vi "MultiSend.vi"() -> ()   [LabVIEW 2019]
uses:
  ByteGSAPIBase/ByteGSAPIBase.lvclass
  TypeDef/ChannelInfo.ctl
  ByteGSAPIBase/LimsTestStep/acquisitions.ctl
  ByteGSAPIBase/UpdateChannelsList/fields.ctl
  <vilib>/Bytelabs/ByteSimpleQ/ByteSimpleQ/ByteSimpleQ.lvlib
panel:
  in  "Start/Stop":bool
  out "Running":bool
  out "error out":errorcluster
  in  "error in (no error)":errorcluster
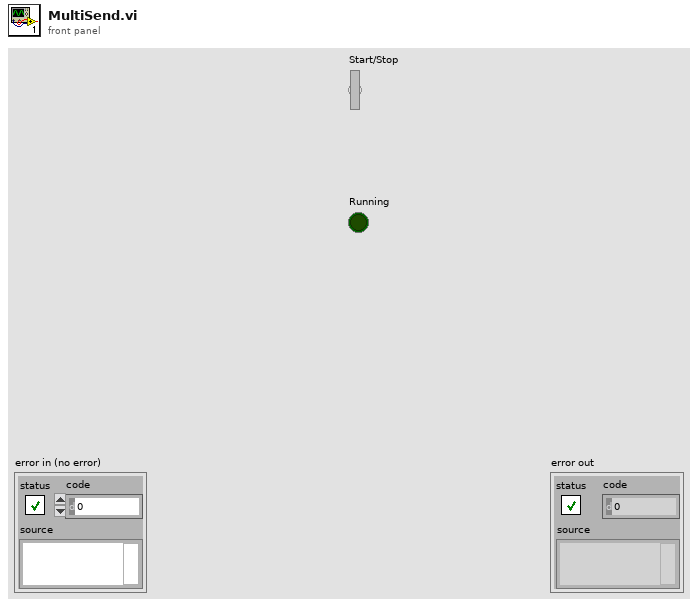
[diagram p1: front panel]
types:
  T1 = typedef "ByteGSWebAPI.lvlib/ByteGSAPIBase.lvclass/acquisitions.ctl" = cluster{"tags":cluster{"step_id":i32, "test_slug":string, "asset_slug":string}, "acquisitions":cluster{"timestamp":string, "fields":cluster{"name":string, "value":dbl}[]}[]}
  T2 = typedef "ChannelInfo.ctl" = cluster{"Tag":string, "HW Resource":string, "Raw":dbl}
  T3 = cluster{"ByteGSAPIBase in":refnum<class "ByteGSAPIBase.lvclass">, "fields":string[][], "Acquisitions":T1, "Info":T2[]}
  T4 = cluster{"ByteGSAPIBase in":refnum<class "ByteGSAPIBase.lvclass">, "queue out":refnum<queue>, "Slug":string, "fields":string[][]}
  T5 = typedef "ByteGSWebAPI.lvlib/ByteGSAPIBase.lvclass/fields.ctl" = cluster{"asset_slug":string, "fields":string[]}
  T6 = cluster{"ByteGSAPIBase out":refnum<class "ByteGSAPIBase.lvclass">, "fields":string[], "Slug":string}
  T7 = cluster{"timestamp":string, "fields":cluster{"name":string, "value":dbl}[]}
  T8 = cluster{"timestamp":string, "fields":cluster{"name":string, "value":dbl}[]}[]
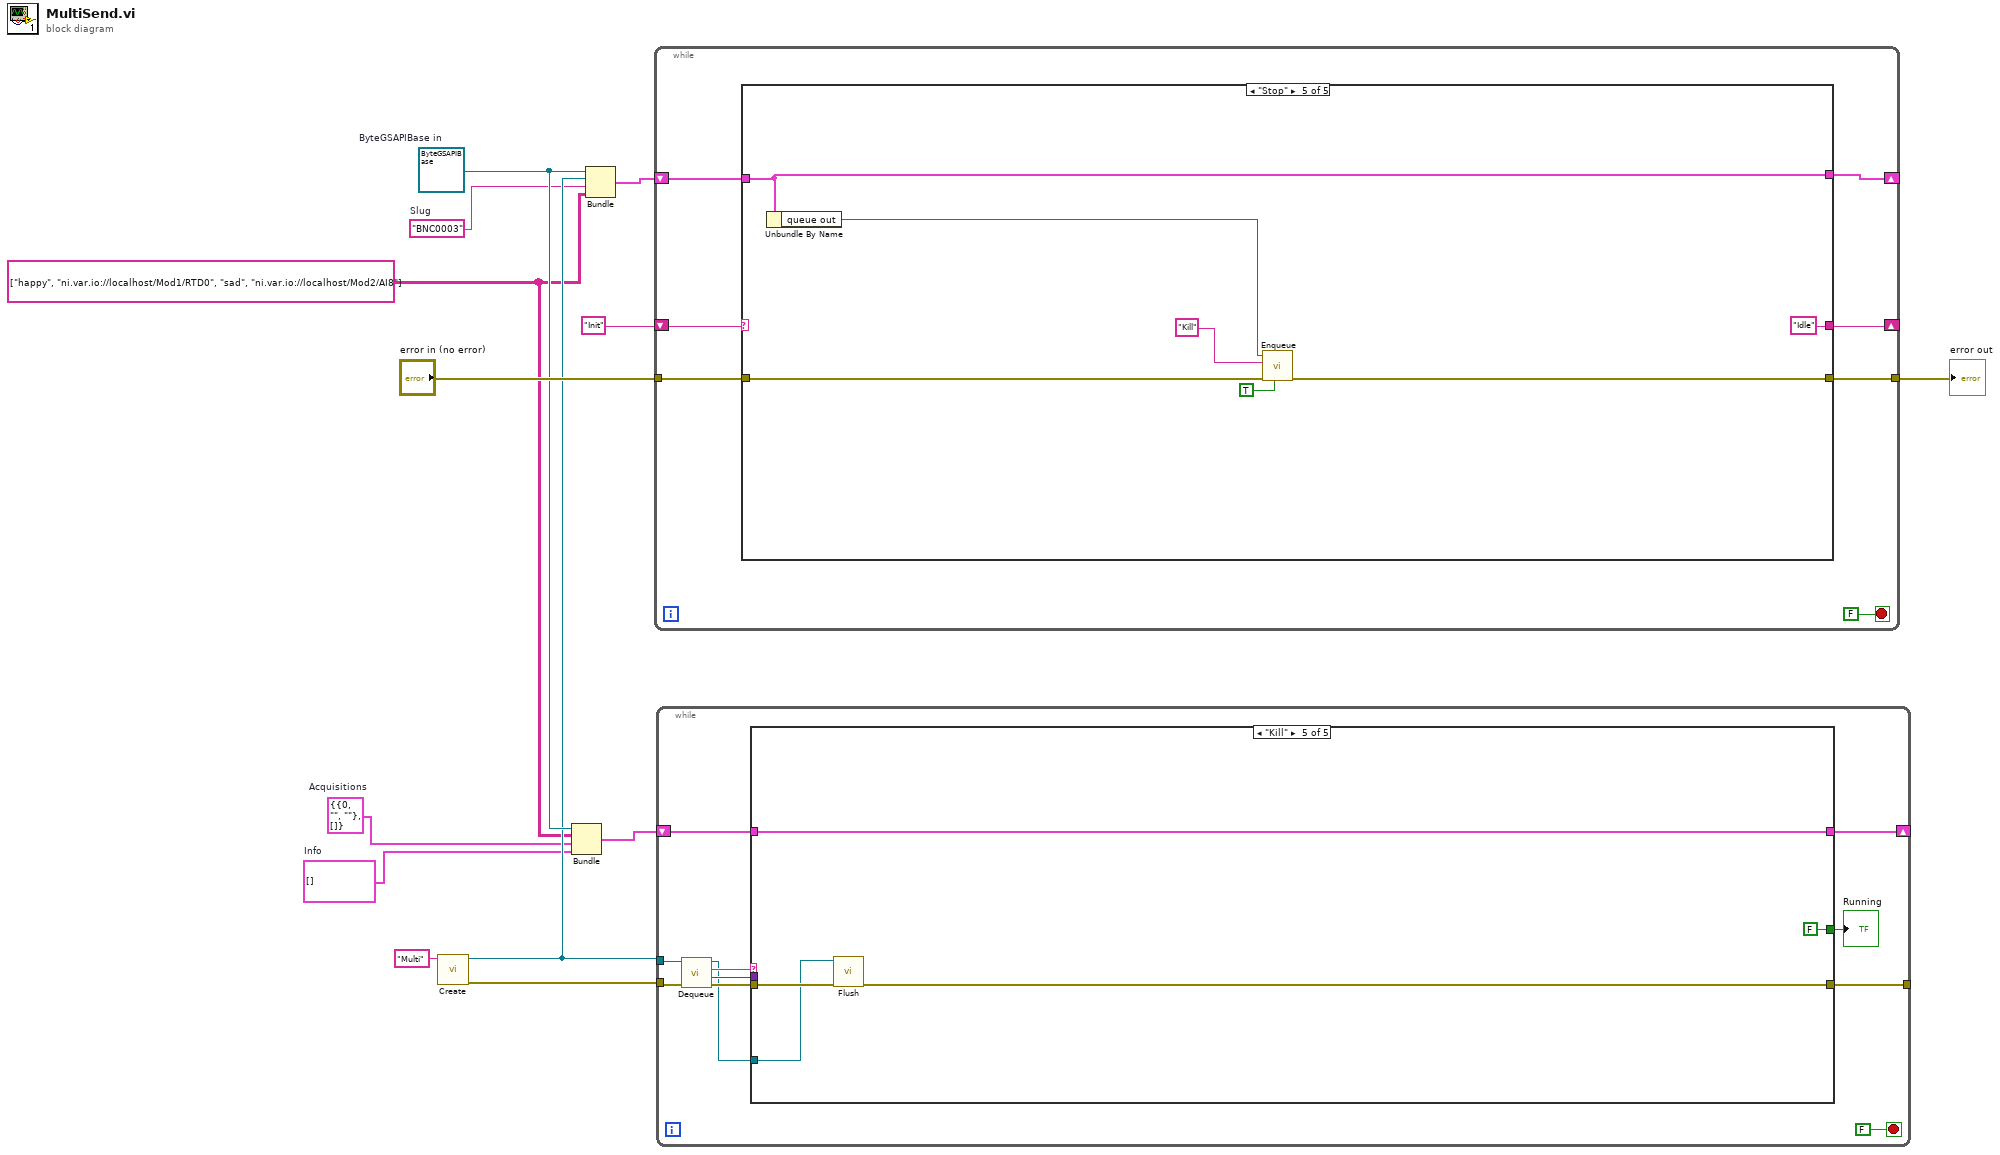
[diagram p0: block diagram]
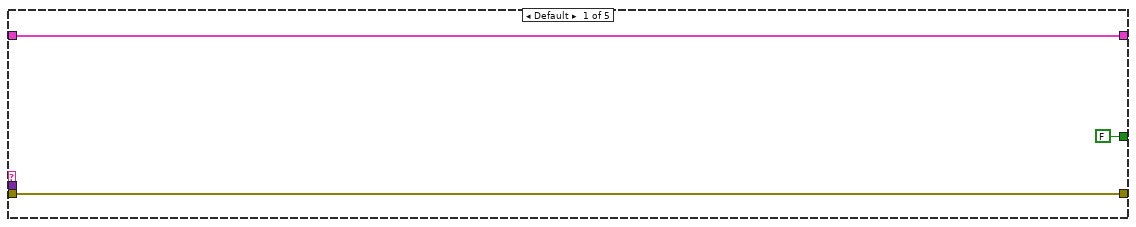
[diagram p2: hidden frame]
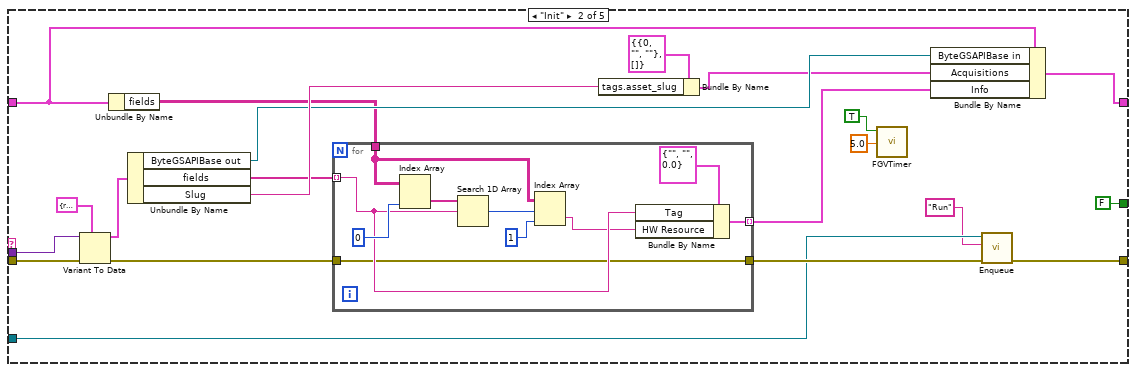
[diagram p3: hidden frame]
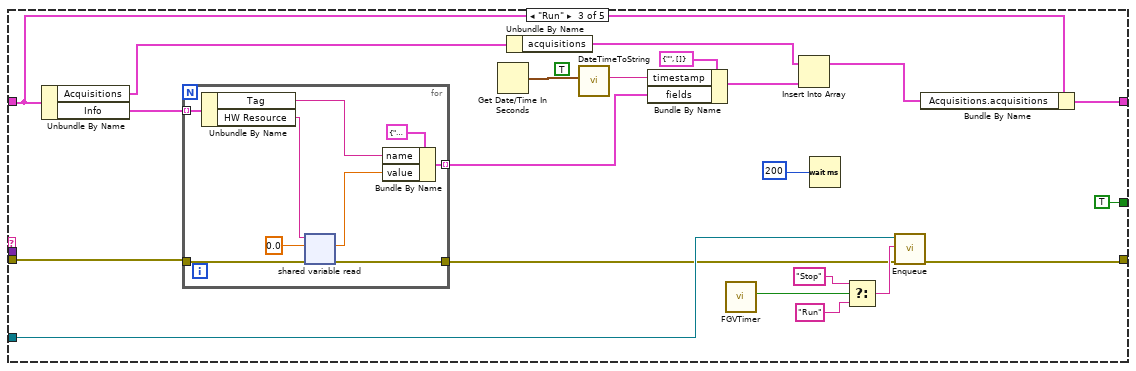
[diagram p4: hidden frame]
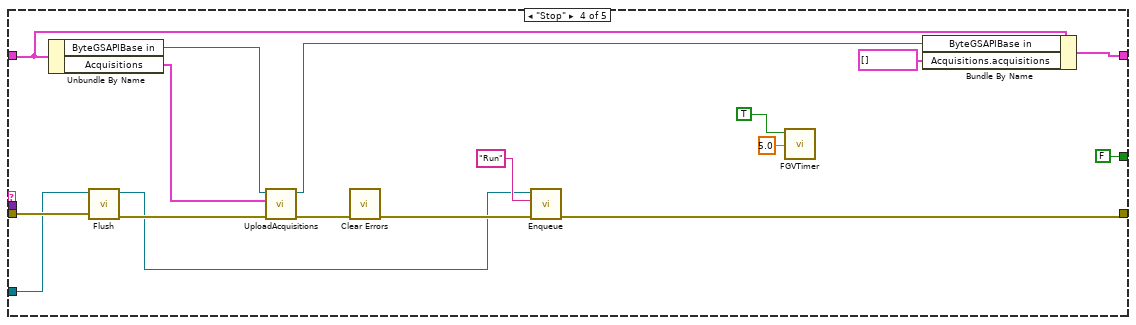
[diagram p5: hidden frame]
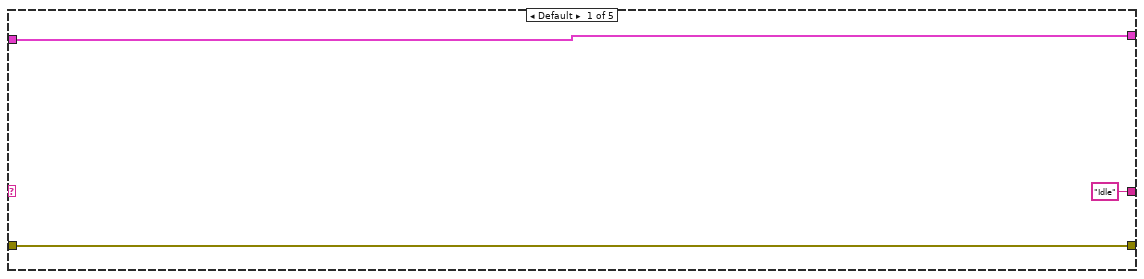
[diagram p6: hidden frame]
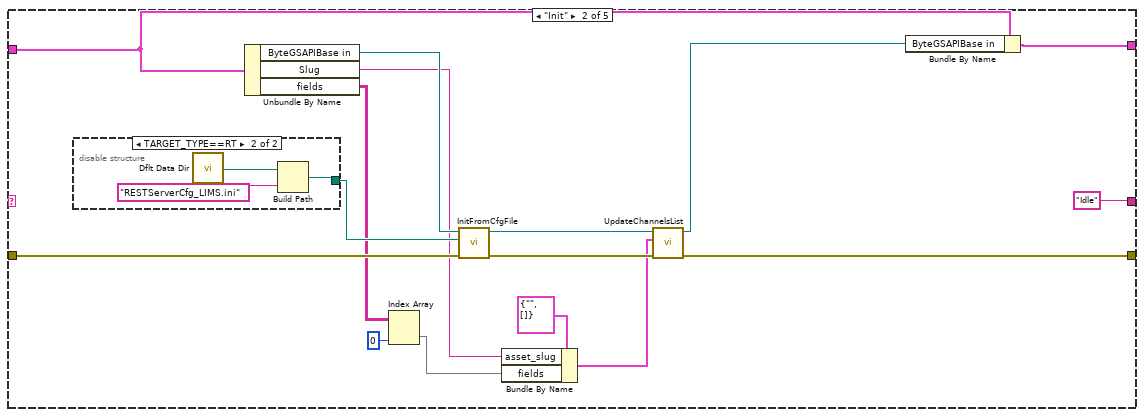
[diagram p7: hidden frame]
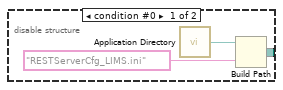
[diagram p8: hidden frame]
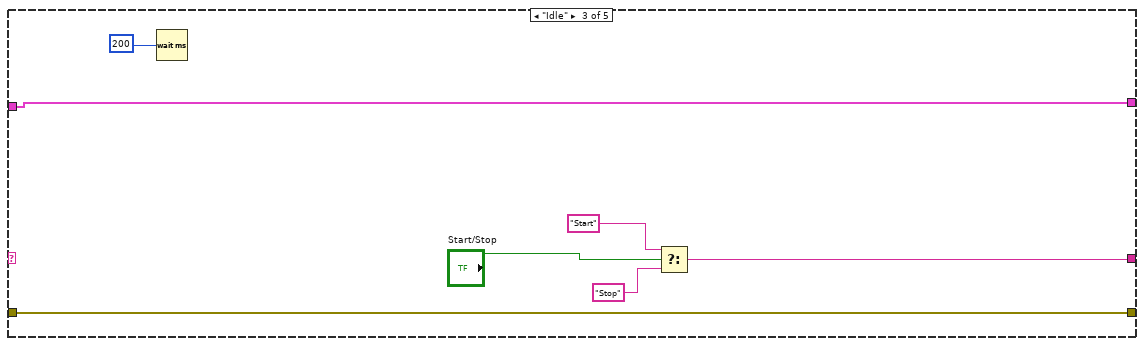
[diagram p9: hidden frame]
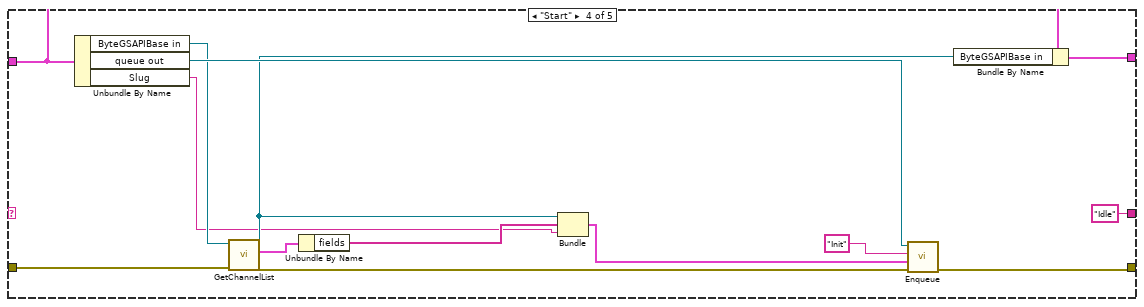
[diagram p10: hidden frame]
diagram:
  w2 = T1 {"tags"={"step_id"=0, "test_slug"="", "asset_slug"=""}, "acquisitions"=[]}  # Acquisitions
  w1 = T2[] []  # Info
  w3 = string[][] [["happy", "ni.var.io://localhost/Mod1/RTD0"], ["sad", "ni.var.io://localhost/Mod2/AI8"]] ("fields")
  w4 = "BNC0003"  # Slug
  w7 = refnum<class "ByteGSAPIBase.lvclass"> refnum  # ByteGSAPIBase in
  n1 = call <vilib>:"Create.vi"("name (unnamed)"="Multi") -> ("error out"=w9:errorcluster, "queue out"=w5:refnum<queue>)  [unwired: 8 in, 1 out]
  n2 = Bundle("ByteGSAPIBase in"=w7, "fields"=w3, "Acquisitions"=w2, "Info"=w1) -> (w6:T3)  [unwired: 1 in]
  n3 = Bundle("ByteGSAPIBase in"=w7, "queue out"=w5, "Slug"=w4, "fields"=w3) -> (w12:T4)  [unwired: 1 in]
  n4 = while {
    shift-right: [w19] -> _
    shift-left: "Init" -> [w20]
    shift-right: [w15] -> _
    shift-left: w12 -> [w18]
    tunnel: "error in (no error)" -> [w17]
    tunnel: [w16] -> w10
    stop <- FALSE stop-if-true
    n5 = case shown="\"Stop\"" w20 {
      tunnel: ["Idle" "Idle" w48 "Idle" "Idle" ("f")] -> w19
      tunnel: w18 -> [w22 w35 w51 w59 w71]
      tunnel: w17 -> [w21 w38 w47 w62 w72]
      tunnel: [w21 w27 w47 w64 w69] -> w16
      tunnel: [w22 w34 w51 w58 w71] -> w15
      frame Default {
      }
      frame "Init" {
        n6 = disable-structure shown="TARGET_TYPE==RT" {
          disable-tunnel: [w40 w43] -> w36
          frame condition #0 {
            n7 = call <vilib>:"Application Directory.vi"() -> ("Application Directory"=w41:path)
            n8 = Build Path(base path=w41, name or relative path="RESTServerCfg_LIMS.ini") -> (appended path=w40:path)
          }
          frame condition #1 (active) {
            n9 = call <vilib>:"Dflt Data Dir.vi"() -> ("App:Default Data Directory"=w45:path)
            n10 = Build Path(base path=w45, name or relative path="RESTServerCfg_LIMS.ini") -> (appended path=w43:path)
          }
        }
        n11 = Unbundle By Name(w35) -> ("ByteGSAPIBase in"=w37:refnum<class "ByteGSAPIBase.lvclass">, "Slug"=w31:string, "fields"=w26:string[][])
        n12 = Index Array(array=w26, index (col)=0 ("disabled index (col)")) -> (element=w24:string[])  [unwired: 1 in]
        n13 = call-dynamic "InitFromCfgFile.vi"("error in (no error)"=w38, "configuration file path"=w36, "ByteGSAPIBase in"=w37) -> ("error out"=w33:errorcluster, "ByteGSAPIBase out"=w29:refnum<class "ByteGSAPIBase.lvclass">)  [unwired: 7 in]
        n14 = Bundle By Name(cluster=T5 {"asset_slug"="", "fields"=[]} ("Channels"), "asset_slug"=w31, "fields"=w24) -> (w30:T5)
        n15 = call "UpdateChannelsList.vi"("error in (no error)"=w33, "Channels"=w30, "ByteGSAPIBase in"=w29) -> ("error out"=w27:errorcluster, "ByteGSAPIBase out"=w28:refnum<class "ByteGSAPIBase.lvclass">)  [unwired: 7 in]
        n16 = Bundle By Name(cluster=w35, "ByteGSAPIBase in"=w28) -> (w34:T4)
      }
      frame "Idle" {
        n17 = Wait (ms)(milliseconds to wait=200) -> ()  [unwired: 1 out]
        n18 = Select(t="Start", s="Start/Stop", f="Stop") -> (s? t:f=w48:string)
      }
      frame "Start" {
        n19 = Unbundle By Name(w59) -> ("ByteGSAPIBase in"=w61:refnum<class "ByteGSAPIBase.lvclass">, "queue out"=w66:refnum<queue>, "Slug"=w55:string)
        n20 = call "GetChannelList.vi"("error in (no error)"=w62, "ByteGSAPIBase in"=w61) -> ("error out"=w53:errorcluster, "Channels"=w60:cluster{"fields":string[]}, "ByteGSAPIBase out"=w56:refnum<class "ByteGSAPIBase.lvclass">)  [unwired: 7 in]
        n21 = Unbundle By Name(w60) -> ("fields"=w57:string[])
        n22 = Bundle("ByteGSAPIBase out"=w56, "fields"=w57, "Slug"=w55) -> (w54:T6)  [unwired: 1 in]
        n23 = call <vilib>:"Enqueue.vi"("error in (no error)"=w53, "data"=w54, "message"="Init", "queue in"=w66) -> ("error out"=w64:errorcluster)  [unwired: 5 in, 2 out]
        n24 = Bundle By Name(cluster=w59, "ByteGSAPIBase in"=w56) -> (w58:T4)
      }
      frame "Stop" {
        n25 = Unbundle By Name(w71) -> ("queue out"=w70:refnum<queue>)
        n26 = call <vilib>:"Enqueue.vi"("High priority (F)"=TRUE, "error in (no error)"=w72, "message"="Kill", "queue in"=w70) -> ("error out"=w69:errorcluster)  [unwired: 5 in, 2 out]
      }
    }
  }
  "error out" <- w10
  n27 = while {
    tunnel: w9 -> [w84]
    tunnel: w5 -> [w83]
    shift-right: [w77] -> _
    shift-left: w6 -> [w78]
    tunnel: [w76] -> _
    stop <- FALSE stop-if-true
    n28 = call <vilib>:"Dequeue.vi"("error in (no error)"=w84, "queue in"=w83) -> ("error out"=w81:errorcluster, "data"=w80:variant, "message"=w79:string, "queue out"=w75:refnum<queue>)  [unwired: 5 in, 1 out]
    n29 = case shown="\"Kill\"" w79 {
      tunnel: w81 -> [w86 w108 w139 w165 w168]
      tunnel: w80 -> [_ w107 _ _ _]
      tunnel: w78 -> [w87 w98 w130 w155 w170]
      tunnel: [w87 w100 w128 w154 w170] -> w77
      tunnel: [w86 w93 w121 w156 w167] -> w76
      tunnel: w75 -> [_ w92 w124 w164 w166]
      tunnel: [FALSE FALSE TRUE FALSE FALSE] -> w74
      frame Default {
      }
      frame "Init" {
        n30 = Variant To Data(error in=w108, type=T6 {"ByteGSAPIBase out"=refnum, "fields"=[], "Slug"=""} ("cluster"), Variant=w107) -> (data=w105:T6, error out=w95:errorcluster)
        n31 = Unbundle By Name(w98) -> ("fields"=w97:string[][])
        n32 = Unbundle By Name(w105) -> ("ByteGSAPIBase out"=w102:refnum<class "ByteGSAPIBase.lvclass">, "fields"=w99:string[], "Slug"=w103:string)
        n33 = for {
          tunnel: w99 -> [w112] mode=indexing
          tunnel: w97 -> [w114]
          tunnel: [w110] -> w96 mode=indexing
          tunnel: w95 -> [w109]
          tunnel: [w109] -> w94
          n34 = Index Array(array=w114, index (col)=0 ("disabled index (col)")) -> (element=w116:string[])  [unwired: 1 in]
          n35 = Search 1D Array(1D array=w116, element=w112) -> (index of element=w115:i32)  [unwired: 1 in]
          n36 = Index Array(array=w114, index (row)=w115, index (col)=1 ("disabled index (col)")) -> (element=w111:string)
          n37 = Bundle By Name(cluster=T2 {"Tag"="", "HW Resource"="", "Raw"=0.0} ("output cluster"), "Tag"=w112, "HW Resource"=w111) -> (w110:T2)
        }
        n38 = Bundle By Name(cluster=T1 {"tags"={"step_id"=0, "test_slug"="", "asset_slug"=""}, "acquisitions"=[]} ("Cluster"), "tags.asset_slug"=w103) -> (w101:T1)
        n39 = call "FGVTimer.vi"("set timer"=5.0, "Reset"=TRUE) -> ()  [unwired: 8 in, 2 out]
        n40 = Bundle By Name(cluster=w98, "ByteGSAPIBase in"=w102, "Acquisitions"=w101, "Info"=w96) -> (w100:T3)
        n41 = call <vilib>:"Enqueue.vi"("error in (no error)"=w94, "message"="Run", "queue in"=w92) -> ("error out"=w93:errorcluster)  [unwired: 6 in, 2 out]
      }
      frame "Run" {
        (unwired) TRUE ("include Time?")
        n42 = Unbundle By Name(w130) -> ("Acquisitions"=w132:T1, "Info"=w138:T2[])
        n43 = for {
          tunnel: w138 -> [w145] mode=indexing
          tunnel: [w141] -> w134 mode=indexing
          tunnel: w139 -> [w148]
          tunnel: [w144] -> w123
          n44 = Unbundle By Name(w145) -> ("Tag"=w142:string, "HW Resource"=w146:string)
          n45 = shared-variable-read(w146, w148, 0.0) -> (w144:errorcluster, w140:dbl)  [unwired: 2 out]
          n46 = Bundle By Name(cluster=cluster{"name":string, "value":dbl} {"name"="", "value"=0.0} ("fields"), "name"=w142, "value"=w140) -> (w141:cluster{"name":string, "value":dbl})
        }
        n47 = Get Date/Time In Seconds() -> (seconds since 1Jan1904=w136:timestamp)
        n48 = Unbundle By Name(w132) -> ("acquisitions"=w131:T8)
        n49 = call "DateTimeToString.vi"("current time"=w136) -> ("date string"=w135:string)  [unwired: 9 in, 1 out]
        n50 = Bundle By Name(cluster=T7 {"timestamp"="", "fields"=[]} ("acquisition"), "timestamp"=w135, "fields"=w134) -> (w133:T7)
        n51 = call "FGVTimer.vi"() -> ("Elapsed?"=w122:bool)  [unwired: 10 in, 1 out]
        n52 = Insert Into Array(array=w131, new element=w133) -> (w129:T8)  [unwired: 1 in]
        n53 = Wait (ms)(milliseconds to wait=200) -> ()  [unwired: 1 out]
        n54 = Select(t="Stop" ("message"), s=w122, f="Run" ("message")) -> (s? t:f=w125:string)
        n55 = call <vilib>:"Enqueue.vi"("error in (no error)"=w123, "message"=w125, "queue in"=w124) -> ("error out"=w121:errorcluster)  [unwired: 6 in, 2 out]
        n56 = Bundle By Name(cluster=w130, "Acquisitions.acquisitions"=w129) -> (w128:T3)
      }
      frame "Stop" {
        n57 = Unbundle By Name(w155) -> ("ByteGSAPIBase in"=w162:refnum<class "ByteGSAPIBase.lvclass">, "Acquisitions"=w161:T1)
        n58 = call <vilib>:"Flush.vi"("error in"=w165, "queue in"=w164) -> ("error out"=w163:errorcluster, "queue out"=w157:refnum<queue>)  [unwired: 8 in]
        n59 = call-dynamic "UploadAcquisitions.vi"("error in (no error)"=w163, "Acquisitions"=w161, "ByteGSAPIBase in"=w162) -> ("error out"=w160:errorcluster, "ByteGSAPIBase out"=w153:refnum<class "ByteGSAPIBase.lvclass">)  [unwired: 7 in]
        n60 = call <vilib>:"Clear Errors.vi"("error in (no error)"=w160) -> ("error out"=w158:errorcluster)  [unwired: 5 in, 1 out]
        n61 = call <vilib>:"Enqueue.vi"("error in (no error)"=w158, "message"="Run", "queue in"=w157) -> ("error out"=w156:errorcluster)  [unwired: 6 in, 2 out]
        n62 = call "FGVTimer.vi"("set timer"=5.0, "Reset"=TRUE) -> ()  [unwired: 8 in, 2 out]
        n63 = Bundle By Name(cluster=w155, "ByteGSAPIBase in"=w153, "Acquisitions.acquisitions"=T8 []) -> (w154:T3)
      }
      frame "Kill" {
        n64 = call <vilib>:"Flush.vi"("error in"=w168, "queue in"=w166) -> ("error out"=w167:errorcluster)  [unwired: 8 in, 1 out]
      }
    }
    "Running" <- w74
  }
